vi "InspectTell.vi"(6 "Error":errorcluster, 7 "Actor":refnum<class "Actor Layer.lvclass">, 10 "Msg":T10 {"Msg Attribs"."Listen Absolute Time" format="%<%x %.3X>T"; "Msg Attribs"."Tell Absolute Time" format="%<%x %.3X>T"}, 11 "Actor":T1) -> (1 "Tell":bool=TRUE, 2 "Msg":T10 {"Msg Attribs"."Listen Absolute Time" format="%<%x %.3X>T"; "Msg Attribs"."Tell Absolute Time" format="%<%x %.3X>T"}, 3 "Actor":T1, 4 "Error":errorcluster, 5 "Actor":refnum<class "Actor Layer.lvclass">)   [LabVIEW 2020, in "_Template.lvlib" / "{{Actor}}.lvlib" / "Actor Layer.lvclass"]
uses:
  Actor Layer.lvclass
  Actor Layer.lvclass/Actor Layer.ctl
  jettl/jettl/Actor Layer/Actor Layer.lvclass
  jettl/jettl/Msg/Msg.lvclass
  jettl/jettl/Origin.ctl
  jettl/jettl/jettl.lvlib
  jettl/jettl/Msg Attribs.ctl
  jettl/jettl/Lifecycle.ctl
  jettl/jettl/Msg.ctl
  jettl/jettl/Post Setup.ctl
  jettl/jettl/Pre Setup.ctl
  jettl/jettl/Msg Set.ctl
  jettl/jettl/Actor Attribs.ctl
  jettl/jettl/Children.ctl
  jettl/jettl/Actor.ctl
  jettl/jettl/Layer Type.ctl
  jettl/jettl/Layer Attribs.ctl
  jettl/jettl/Layer Map.ctl
  jettl/jettl/Implemented Map.ctl
panel:
  # "This front panel should not be manipulated."
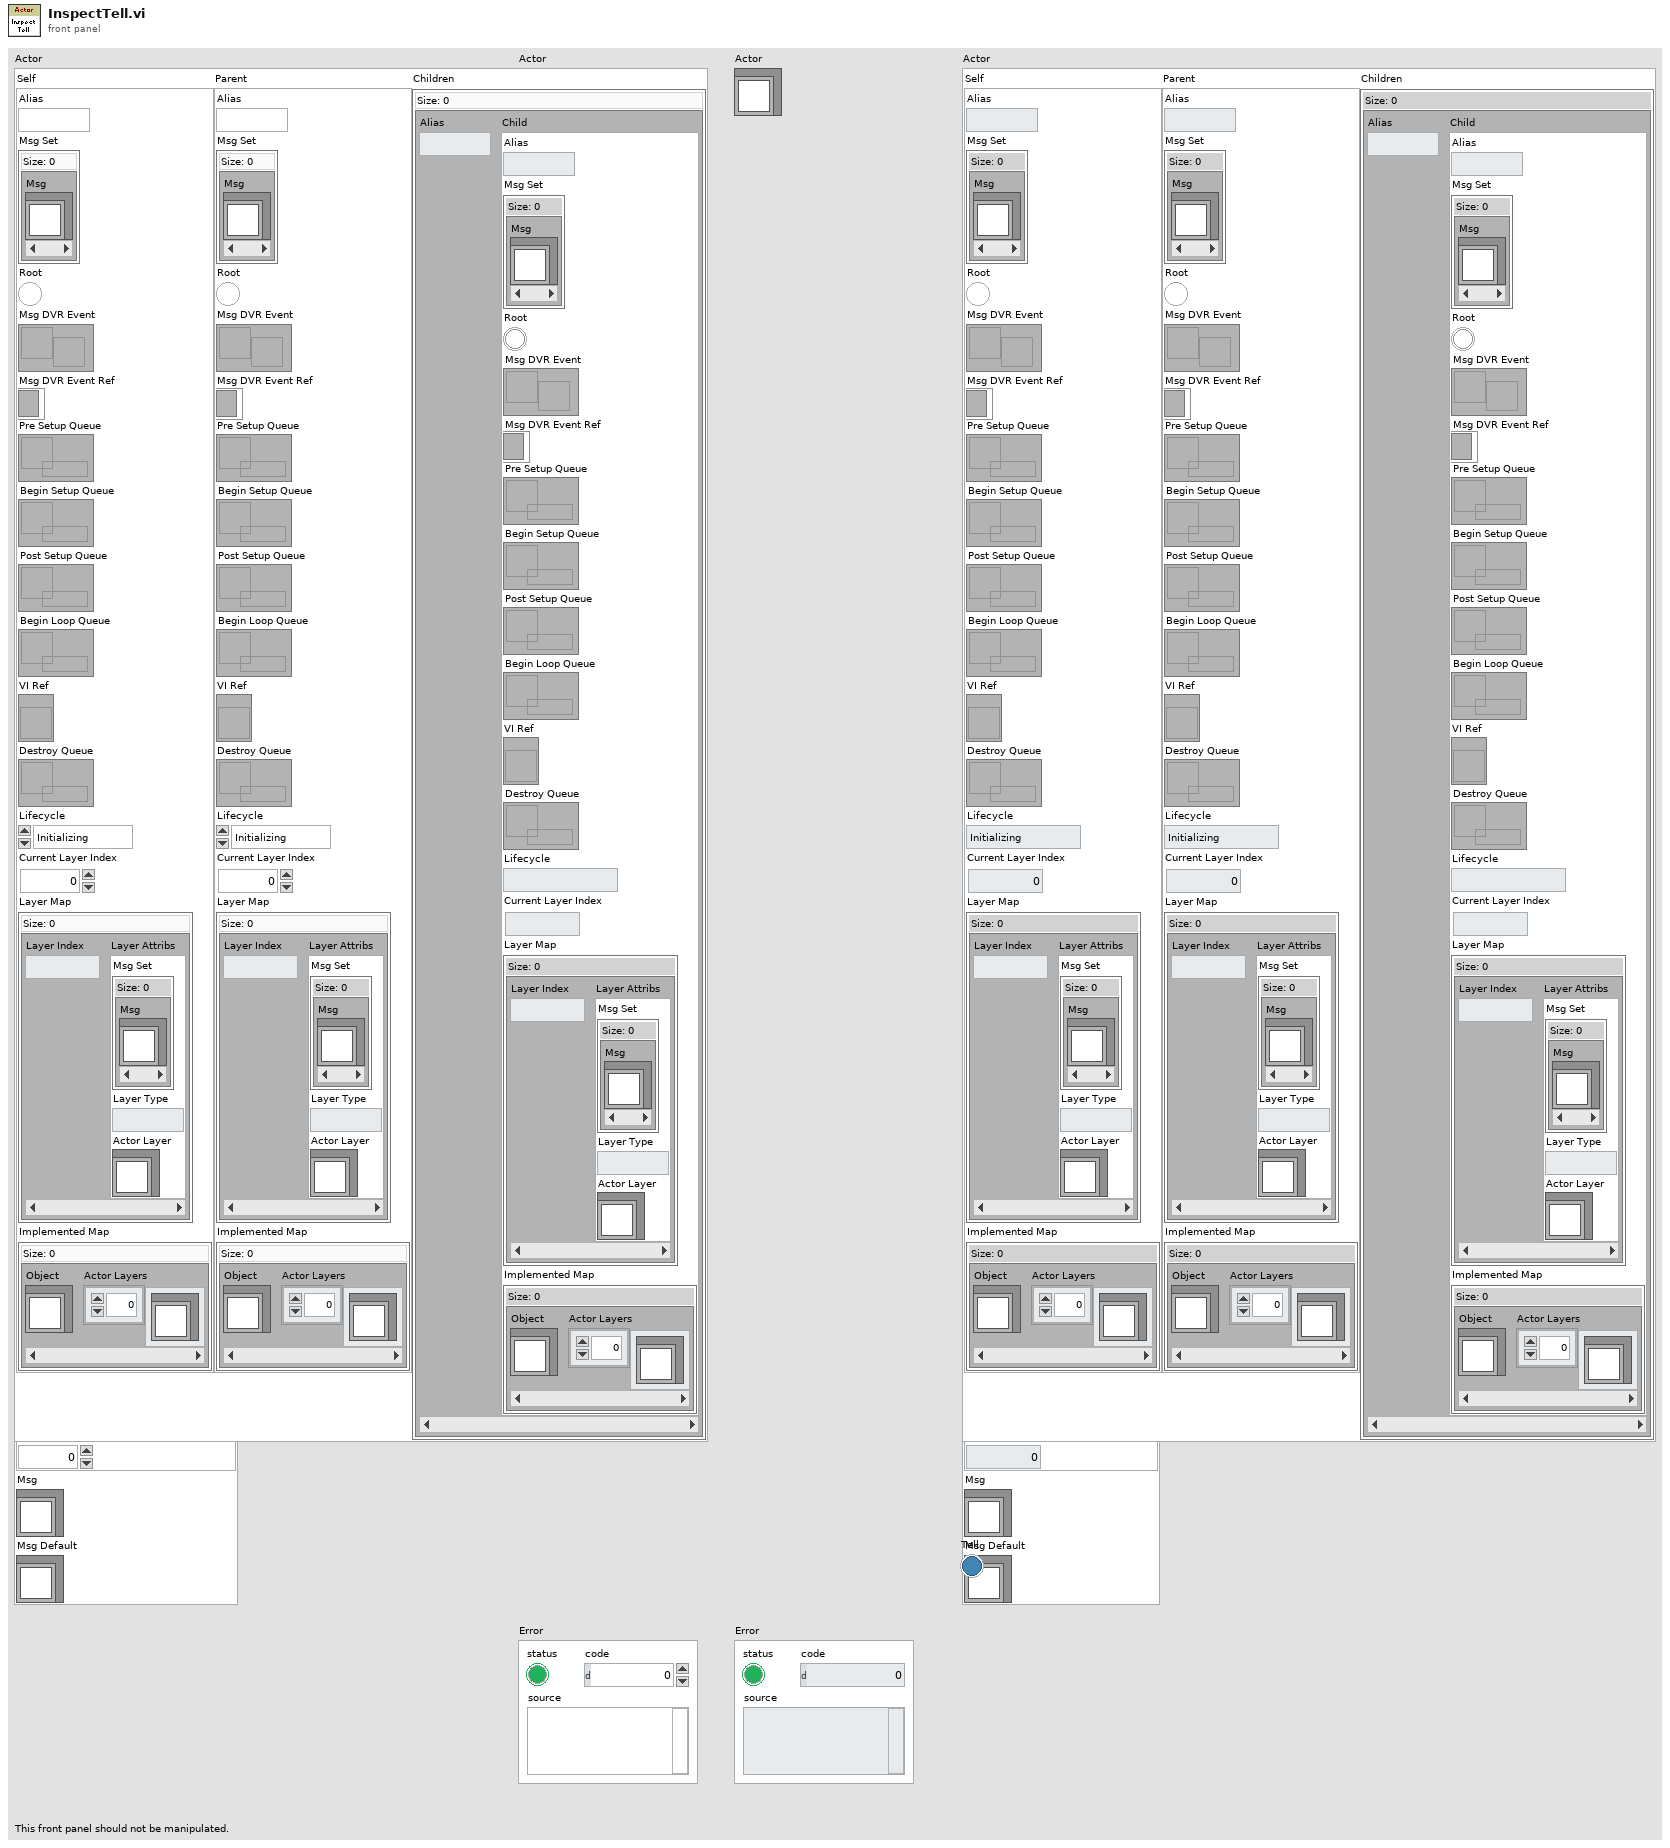
[diagram p1: front panel]
types:
  T1 = typedef "jettl.lvlib/Actor.ctl" = cluster{"Self":T2, "Parent":T2, "Children":T9}
  T2 = typedef "jettl.lvlib/Actor Attribs.ctl" = cluster{"Alias":string, "Msg Set":T3, "Root":bool, "Msg DVR Event":refnum<user-event>, "Msg DVR Event Ref":refnum<event-registration>, "Pre Setup Queue":refnum<queue>, "Begin Setup Queue":refnum<queue>, "Post Setup Queue":refnum<queue>, "Begin Loop Queue":refnum<queue>, "VI Ref":refnum<vi>, "Destroy Queue":refnum<queue>, "Lifecycle":T4, "Current Layer Index":i32, "Layer Map":T5, "Implemented Map":T8}
  T3 = typedef "jettl.lvlib/Msg Set.ctl" = set{refnum<class "Msg.lvclass">}
  T4 = typedef "jettl.lvlib/Lifecycle.ctl" = enum16{"Initializing", "Setting Up", "Starting", "Running", "Stopping", "Tearing Down", "Terminated"}
  T5 = typedef "jettl.lvlib/Layer Map.ctl" = map{i32, T6}
  T6 = typedef "jettl.lvlib/Layer Attribs.ctl" = cluster{"Msg Set":T3, "Layer Type":T7, "Actor Layer":refnum<class "Actor Layer.lvclass">}
  T7 = typedef "jettl.lvlib/Layer Type.ctl" = enum16{"Base", "InnerGlobal", "InnerLocal", "Outer"}
  T8 = typedef "jettl.lvlib/Implemented Map.ctl" = map{refnum<class>, refnum<class "Actor Layer.lvclass">[]}
  T9 = typedef "jettl.lvlib/Children.ctl" = map{string, T2}
  T10 = typedef "jettl.lvlib/Msg.ctl" = cluster{"Msg Attribs DVR":refnum<data-value>, "Msg Attribs":T11, "Msg":refnum<class "Msg.lvclass">, "Msg Default":refnum<class "Msg.lvclass">}
  T11 = typedef "jettl.lvlib/Msg Attribs.ctl" = cluster{"Priority":bool, "Listener Alias":string, "Teller Alias":string, "Teller Lifecycle":T4, "Teller Origin":T12, "Tell Absolute Time":timestamp, "Tell Relative Time":dbl, "Listen Absolute Time":timestamp, "Listen Relative Time":dbl}
  T12 = typedef "jettl.lvlib/Origin.ctl" = enum16{"Self", "Parent", "Child"}
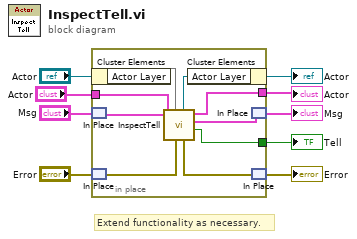
[diagram p0: block diagram]
diagram:
  # "Extend functionality as necessary."
  n1 = in-place {
    in-place-border: [w12] -> w3
    in-place-border: "Actor" -> [w14]
    in-place-border: [w13] -> w1
    n2 = in-place-cluster #1("Actor") -> ("Actor Layer"=w18)
    n3 = in-place-match #2("Msg") -> (w10:T10)
    n4 = in-place-match #3("Error") -> (w16:errorcluster)
    n5 = call-dynamic "InspectTell.vi"("Error"=w16, 7:"Actor"=w18, "Msg"=w10, 11:"Actor"=w14) -> ("Tell"=w12:bool, "Msg"=w11:T10, 3:"Actor"=w13:T1, "Error"=w15:errorcluster, 5:"Actor"=w17:refnum<class "Actor Layer.lvclass">)  [unwired: 3 in]
    n6 = in-place-cluster #1("Actor Layer"=w17) -> (→"Actor":refnum<class "Actor Layer.lvclass">)
    n7 = in-place-match #2(w11) -> (→"Msg":T10)
    n8 = in-place-match #3(w15) -> (→"Error":errorcluster)
  }
  "Tell" <- w3
  "Actor" <- w1
